vi "IntakeBeamBreakGetState.vi"() -> (2 "Switch Pressed":bool)   [LabVIEW 2014, in "IntakeLib.lvlib"]
uses:
  IntakeLib.lvlib
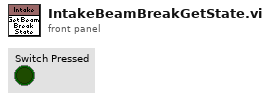
[diagram p1: front panel]
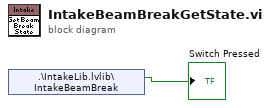
[diagram p0: block diagram]
diagram:
  n1 = shared-variable ".\\IntakeLib.lvlib\\IntakeBeamBreak"() -> (→"Switch Pressed":bool)  [unwired: 1 in, 1 out]
